vi "Scan engine status.vi"(7 "Actions":T3=enum."Clear", 8 "Error In":errorcluster, 9 "Current state in":T2=enum."Init(GPU FFT)", 10 "Status in":T1 {"Previous cut plane" format="%#_13g"; "Current image plane" format="%#_13g"}, 11 "XY Graph in":cluster{"X":dbl, "Y":dbl}[](graph)) -> (0 "Error Out":errorcluster, 1 "Current state out":T2=enum."Init(GPU FFT)", 2 "Status out":T1 {"Previous cut plane" format="%#_13g"; "Current image plane" format="%#_13g"}, 3 "XY Graph out":cluster{"X":dbl, "Y":dbl}[](graph))   [LabVIEW 2018]
uses:
  Controls/Go Scan Actions.ctl
  Controls/FGV Actions.ctl
  type defines/Status cluster.ctl
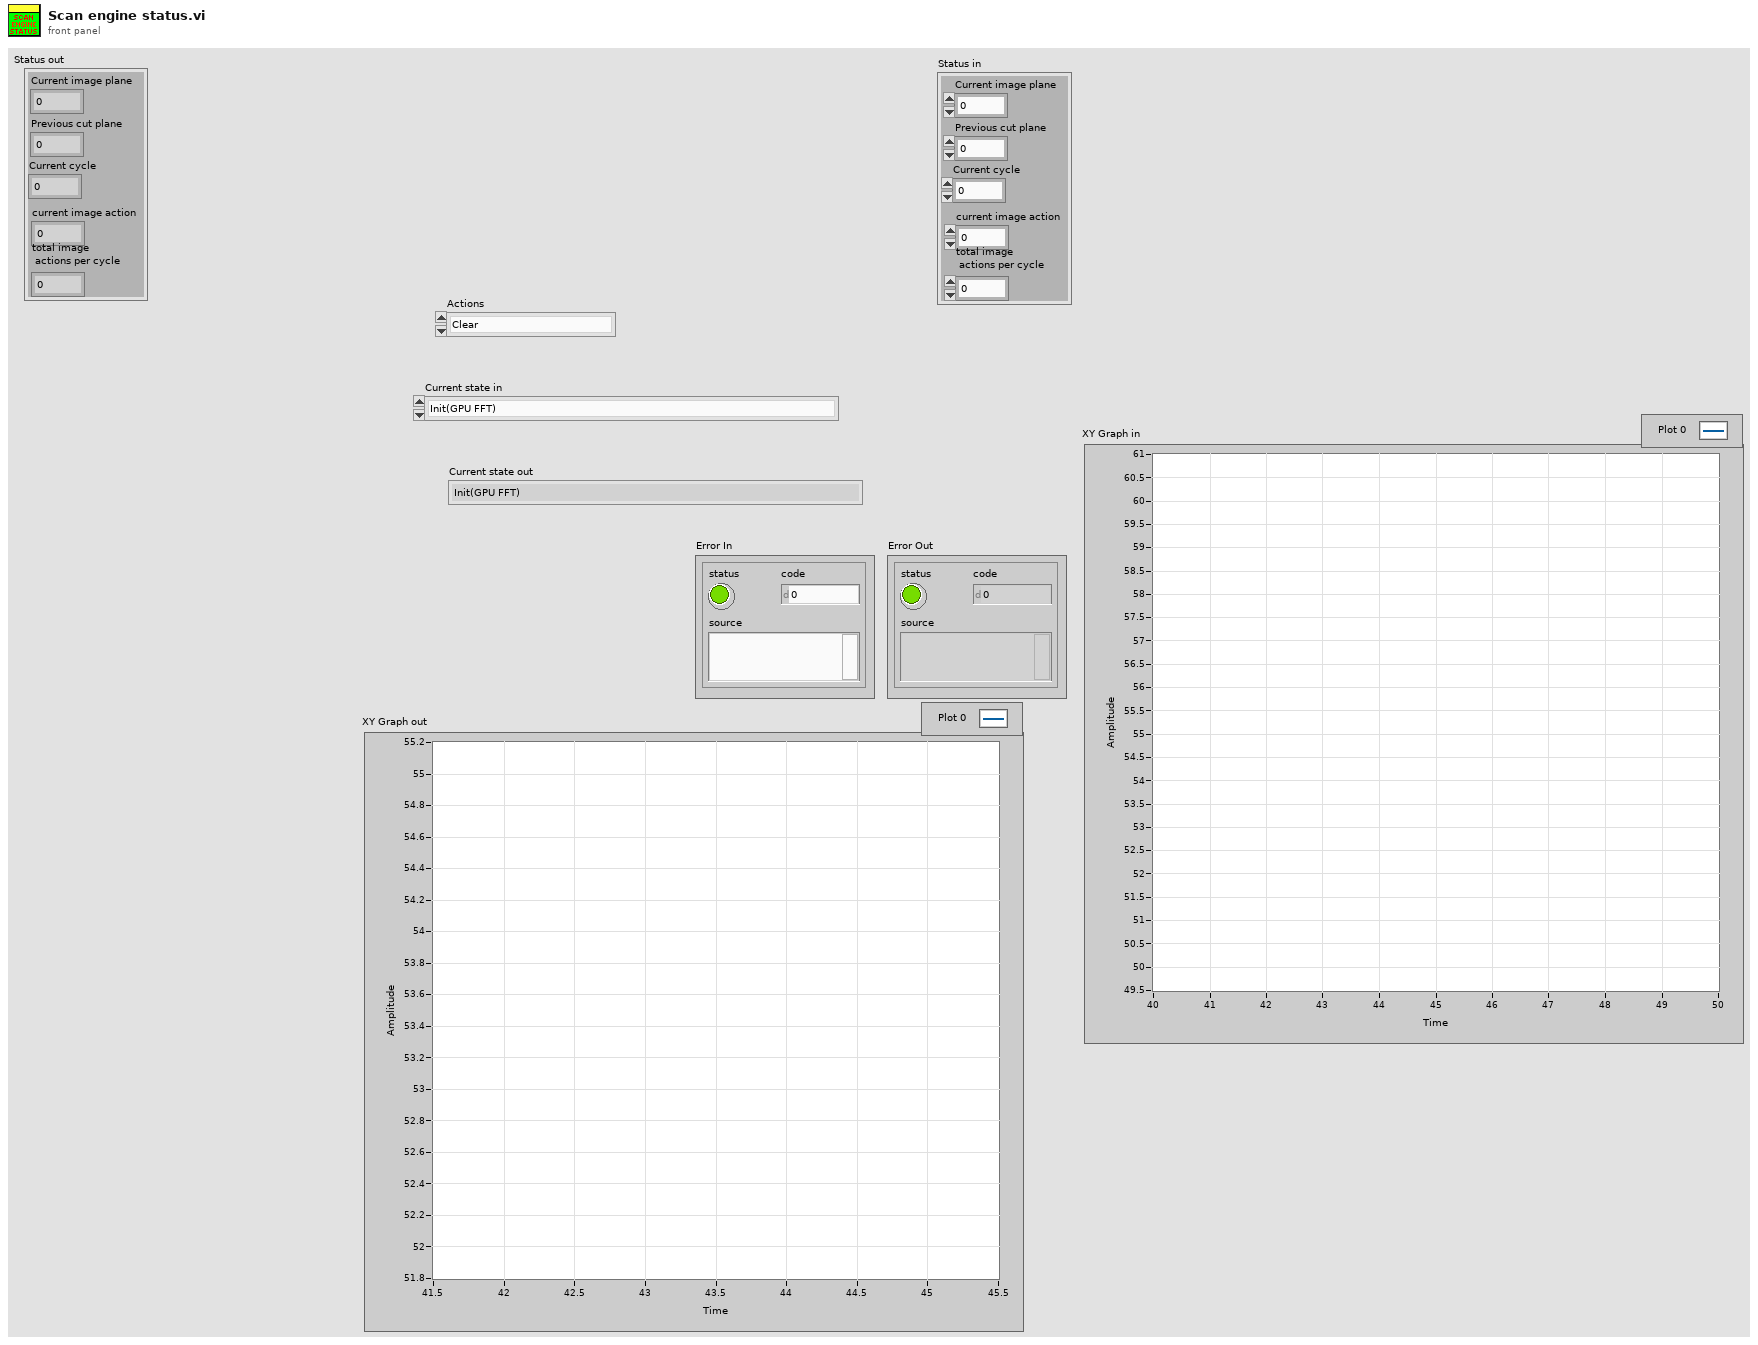
[diagram p1: front panel]
types:
  T1 = typedef "Status cluster.ctl" = cluster{"Current image plane":dbl, "Previous cut plane":dbl, "Current cycle":dbl, "current image action":dbl, "total image\n actions per cycle":dbl}
  T2 = typedef "Go Scan Actions.ctl" = enum16{"Init(ThorOCT Spatial)", "Init(ThorOCT Spectral)", "Init(GPU FFT)", "Init(Alazar FFT)", "Init Scan Head(ThorOCT Spectral)", "Init Scan Head(ThorOCT Spatial)", "Init Scan Head", "Init Table Stage", "Init Vibratome", "Generate Mosaic", "Generate Z Position", "Go to Image Z", "Go Image Home", "Go Mosaic", "Acquire Image(ThorOCT Spatial)", "Acquire Image(ThorOCT Spectral)", "Acquire Image(GPU FFT)", "Acquire Image(Alazar FFT)", "Go Vibratome", "Slice", "Finished(ThorOCT)", "Finished", "Init(Alazar Spectral)", "Frame Start Trigger"}
  T3 = typedef "FGV Actions.ctl" = enum16{"Init", "Set", "Get", "Clear"}
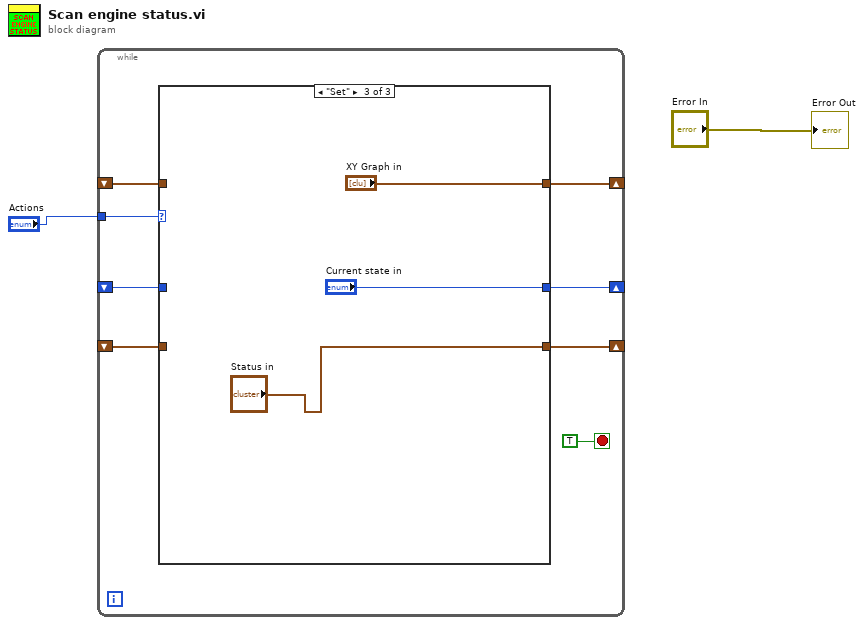
[diagram p0: block diagram]
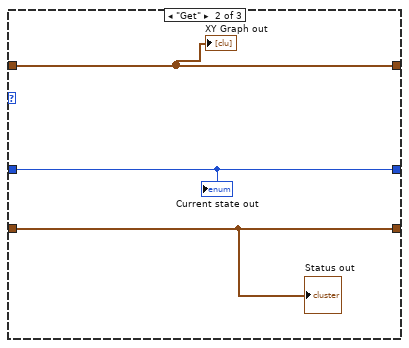
[diagram p3: hidden frame]
diagram:
  n1 = while {
    shift-right: [w10] -> _
    shift-left: _ -> [w7]
    shift-right: [w9] -> _
    shift-left: _ -> [w6]
    tunnel: "Actions" -> [w8]
    shift-right: [w4] -> _
    shift-left: _ -> [w3]
    stop <- TRUE stop-if-true
    n2 = case shown="\"Set\"" w8 {
      tunnel: [_ w12 "XY Graph in"] -> w10
      tunnel: [_ w13 "Current state in"] -> w9
      tunnel: w7 -> [_ w12 _]
      tunnel: w6 -> [_ w13 _]
      tunnel: [_ w11 "Status in"] -> w4
      tunnel: w3 -> [_ w11 _]
      frame "Init", Default {
      }
      frame "Get" {
        "Current state out" <- w13
        "XY Graph out" <- w12
        "Status out" <- w11
      }
      frame "Set" {
      }
    }
  }
  "Error Out" <- "Error In"
